vi "GFITS_LibInit.vi"(4 "totalrows":i32, 5 "namp":i32, 6 "totalcols":i32, 7 "amplifiers":u64, 8 "error in (no error)":errorcluster, 9 "multiple extensions?":bool, 10 "hdutype":i32, 11 "datatype":i32) -> (0 "error out":errorcluster, 2 "return value":i32)   [LabVIEW 2016]
uses:
  c/lib/libgfits.so
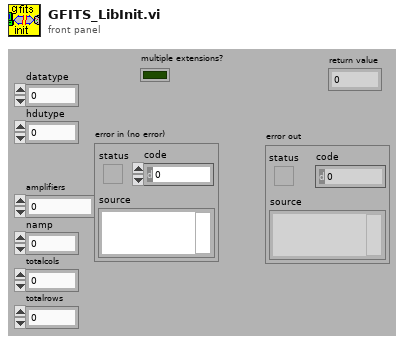
[diagram p1: front panel]
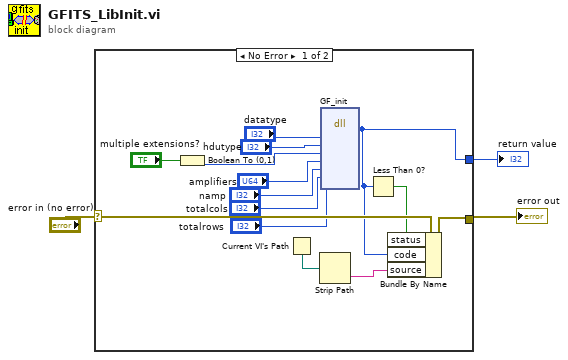
[diagram p0: block diagram]
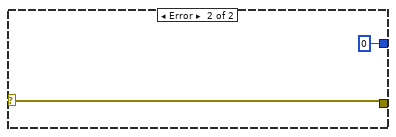
[diagram p2: hidden frame]
diagram:
  n1 = case shown="No Error" "error in (no error)" {
    selector: "error in (no error)" -> [w17 w19]
    tunnel: [w15 0] -> w3
    tunnel: [w12 w19] -> w1
    frame No Error {
      n2 = Boolean To (0,1)(Boolean="multiple extensions?") -> (0, 1=w4:i16)
      n3 = Current VI's Path() -> (path=w14:path)
      n4 = Strip Path(path=w14) -> (name=w13:string)  [unwired: 1 out]
      n5 = dll-call lib="home/simager/panview/PAN/Modules/GFITS/private/c/lib/libgfits.so" fn="GF_init"("datatype"="datatype", "hdutype"="hdutype", "mult"=w4, "amplifiers"="amplifiers", "namp"="namp", "totalcols"="totalcols", "totalrows"="totalrows") -> ("return type"=w15:i32)  [unwired: 9 in, 3 out]
      n6 = Less Than 0?(x=w15) -> (x < 0?=w16:bool)
      n7 = Bundle By Name(cluster=w17, "status"=w16, "code"=w15, "source"=w13) -> (w12:errorcluster)
    }
    frame Error {
    }
  }
  "return value" <- w3
  "error out" <- w1
